vi "Search Bookmarks with event names.vi"(6 "Round Trip Name (Broadcast":string, 8 "error in":errorcluster, 9 "Event Name":string, 10 "VIs to Search for Bookmarks Paths":path[](array[path]), 11 "Application in":refnum<vi>) -> (0 "error out":errorcluster)   [LabVIEW 2016, in "PantherLAB_Scripting.lvlib"]
uses:
  PantherLAB_Scripting.lvlib
  <vilib>/Utility/traverseref.llb/TRef TravTarget.ctl
  <vilib>/Utility/traverseref.llb/VI Scripting - Traverse.lvlib
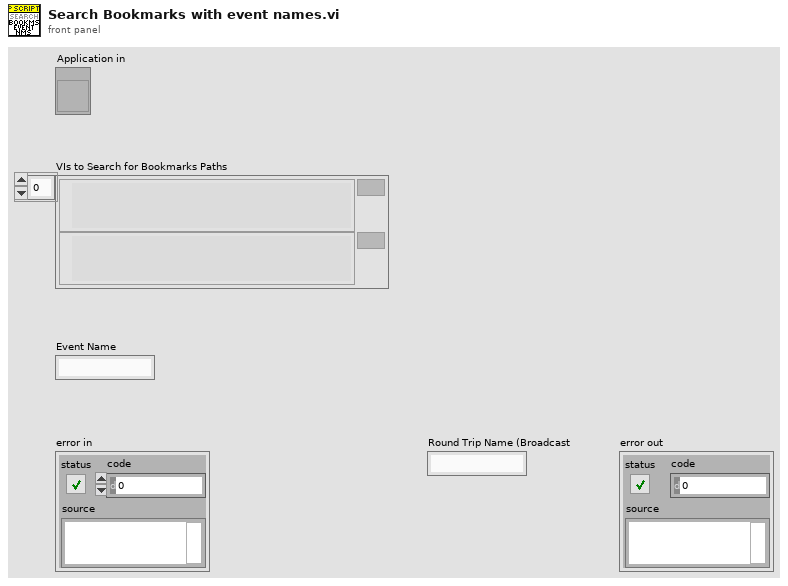
[diagram p1: front panel]
types:
  T1 = typedef "TRef TravTarget.ctl" = enum16{"FP", "BD", "Other"}
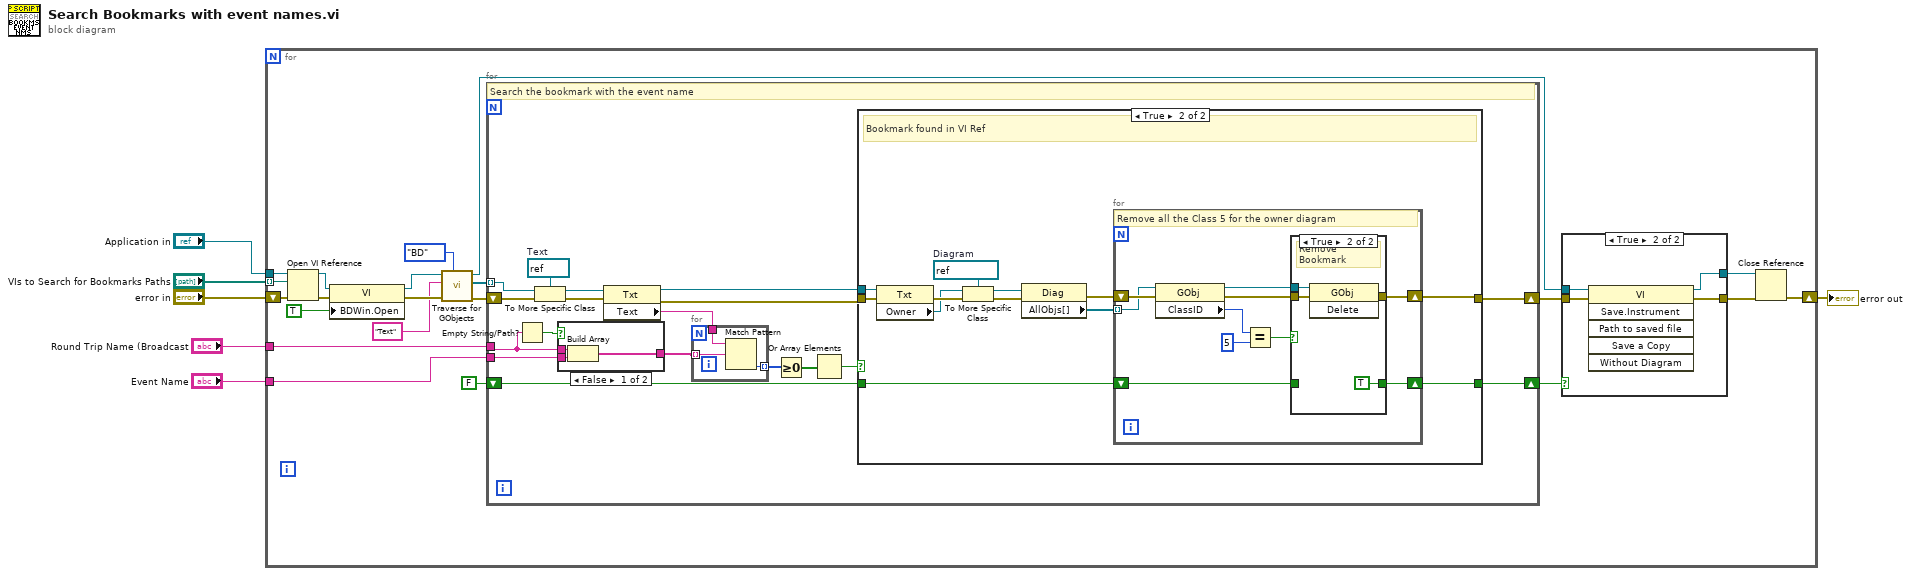
[diagram p0: block diagram]
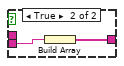
[diagram p4: hidden frame]
diagram:
  n1 = for {
    tunnel: "Application in" -> [w15]
    tunnel: "Event Name" -> [w13]
    tunnel: "VIs to Search for Bookmarks Paths" -> [w12] mode=indexing
    shift-right: [w22] -> w6
    shift-left: "error in" -> [w23]
    tunnel: "Round Trip Name (Broadcast" -> [w7]
    n2 = Open VI Reference(application reference (local)=w15, vi path=w12, error in (no error)=w23) -> (vi reference=w17:refnum<vi>, error out=w25:errorcluster)  [unwired: 3 in]
    n3 = property class="VI"(reference=w17, error in=w25, "BDWin.Open"=TRUE ("Block Diagram Window:Open")) -> (reference out=w16:refnum<vi>, error out=w24:errorcluster)
    n4 = call <vilib>:"Traverse for GObjects.vi"("Traverse Target"=TRef_TravTarget."BD", "error in (no error)"=w24, "Class Name"="Text", "VI Refnum"=w16) -> ("error out"=w27:errorcluster, "References"=w14:refnum<vi>[], "dup VI Refnum"=w10:refnum<vi>)  [unwired: 4 in, 1 out]
    n5 = for {
      shift-right: [w44] -> w26
      shift-left: w27 -> [w45]
      tunnel: w14 -> [w40] mode=indexing
      tunnel: w13 -> [w37]
      shift-right: [w34] -> w8
      shift-left: FALSE -> [w35]
      tunnel: w7 -> [w29]
      w41 = refnum<vi> refnum  # Text
      # "Search the bookmark with the event name"
      n6 = Empty String/Path?(string/path=w29) -> (empty?=w28:bool)
      n7 = To More Specific Class(target class=w41, reference=w40, error in=w45) -> (specific class reference=w39:refnum<vi>, error out=w43:errorcluster)
      n8 = case shown="False" w28 {
        tunnel: w37 -> [w78 w80]
        tunnel: [w77 w79] -> w33
        tunnel: w29 -> [w76 _]
        frame False {
          n9 = Build Array(w76, w78) -> (w77:string[])
        }
        frame True {
          n10 = Build Array(w80) -> (w79:string[])
        }
      }
      n11 = property class="Txt"(reference=w39, error in=w43) -> (reference out=w36:refnum<vi>, error out=w42:errorcluster, "Text"=w38:string)
      n12 = for {
        tunnel: w38 -> [w83]
        tunnel: [w82] -> w32 mode=indexing
        tunnel: w33 -> [w81] mode=indexing
        n13 = Match Pattern(string=w83, regular expression=w81) -> (offset past match=w82:i32)  [unwired: 1 in, 3 out]
      }
      n14 = Greater Or Equal To 0?(x=w32) -> (x >= 0?=w31:bool[])
      n15 = Or Array Elements(Boolean array=w31) -> (logical OR=w30:bool)
      n16 = case shown="True" w30 {
        tunnel: w42 -> [w47 w59]
        tunnel: w36 -> [_ w54]
        tunnel: [w47 w58] -> w44
        tunnel: w35 -> [w46 w53]
        tunnel: [w46 w52] -> w34
        frame False {
          # "Text Not Found"
        }
        frame True {
          w50 = refnum<vi> refnum  # Diagram
          # "Bookmark found in VI Ref"
          n17 = property class="Txt"(reference=w54, error in=w59) -> (error out=w57:errorcluster, "Owner"=w51:refnum<vi>)  [unwired: 1 out]
          n18 = To More Specific Class(target class=w50, reference=w51, error in=w57) -> (specific class reference=w48:refnum<vi>, error out=w55:errorcluster)
          n19 = property class="Diag"(reference=w48, error in=w55) -> (error out=w56:errorcluster, "AllObjs[]"=w49:refnum<vi>[])  [unwired: 1 out]
          n20 = for {
            tunnel: w49 -> [w66] mode=indexing
            shift-right: [w67] -> w58
            shift-left: w56 -> [w69]
            shift-right: [w60] -> w52
            shift-left: w53 -> [w61]
            # "Remove all the Class 5 for the owner diagram"
            n21 = property class="GObj"(reference=w66, error in=w69) -> (reference out=w62:refnum<vi>, error out=w68:errorcluster, "ClassID"=w65:u32)
            n22 = Equal?(x=w65, y=u32 5) -> (x = y?=w63:bool)
            n23 = case shown="True" w63 {
              tunnel: w68 -> [w71 w75]
              tunnel: w62 -> [_ w73]
              tunnel: [w71 w74] -> w67
              tunnel: w61 -> [w70 _]
              tunnel: [w70 TRUE] -> w60
              frame False {
              }
              frame True {
                # "Remove Bookmark"
                n24 = invoke class="GObj" method="Delete"(reference=w73, error in=w75) -> (error out=w74:errorcluster)  [unwired: 1 in, 2 out]
              }
            }
          }
        }
      }
    }
    n25 = case shown="True" w8 {
      tunnel: w26 -> [w85 w89]
      tunnel: [w85 w88] -> w21
      tunnel: w10 -> [w84 w87]
      tunnel: [w84 w86] -> w9
      frame False {
      }
      frame True {
        n26 = invoke class="VI" method="Save.Instrument"(reference=w87, error in=w89) -> (reference out=w86:refnum<vi>, error out=w88:errorcluster)  [unwired: 4 in, 4 out]
      }
    }
    n27 = Close Reference(reference=w9, error in (no error)=w21) -> (error out=w22:errorcluster)
  }
  "error out" <- w6
